vi "PID.vi"(6 "Reset I?":bool, 7 "permissable error range":dbl, 9 "Loop Period":dbl, 10 "Gains":cluster{"kP":dbl, "kI":dbl, "kD":dbl}, 11 "Error":dbl format="%#_13g") -> (1 "PID Variables":cluster{"P":dbl, "I":dbl, "D":dbl, "P+I+D":dbl}, 2 "Device has arrived":bool, 3 "Output":dbl)   [LabVIEW 2015]
uses:
  <vilib>/Analysis/3filter.llb/Filter Passband Type.ctl
  <vilib>/ptbypt/NI_PtbyPt.lvlib
  <vilib>/Analysis/NI_AALBase.lvlib
panel:
  in  "I_Cap":dbl=1.0
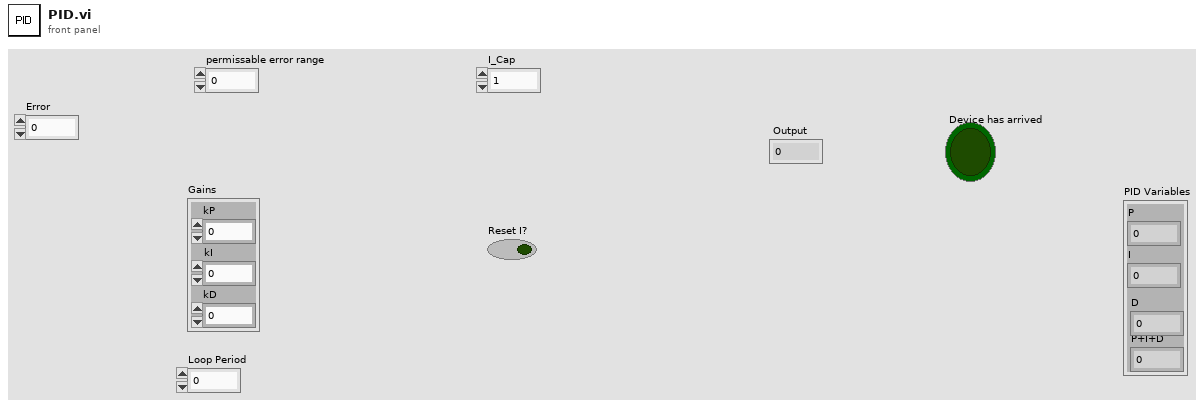
[diagram p1: front panel]
types:
  T1 = typedef "NI_AALBase.lvlib/Filter Passband Type.ctl" = enum32{"Lowpass", "Highpass", "Bandpass", "Bandstop"}
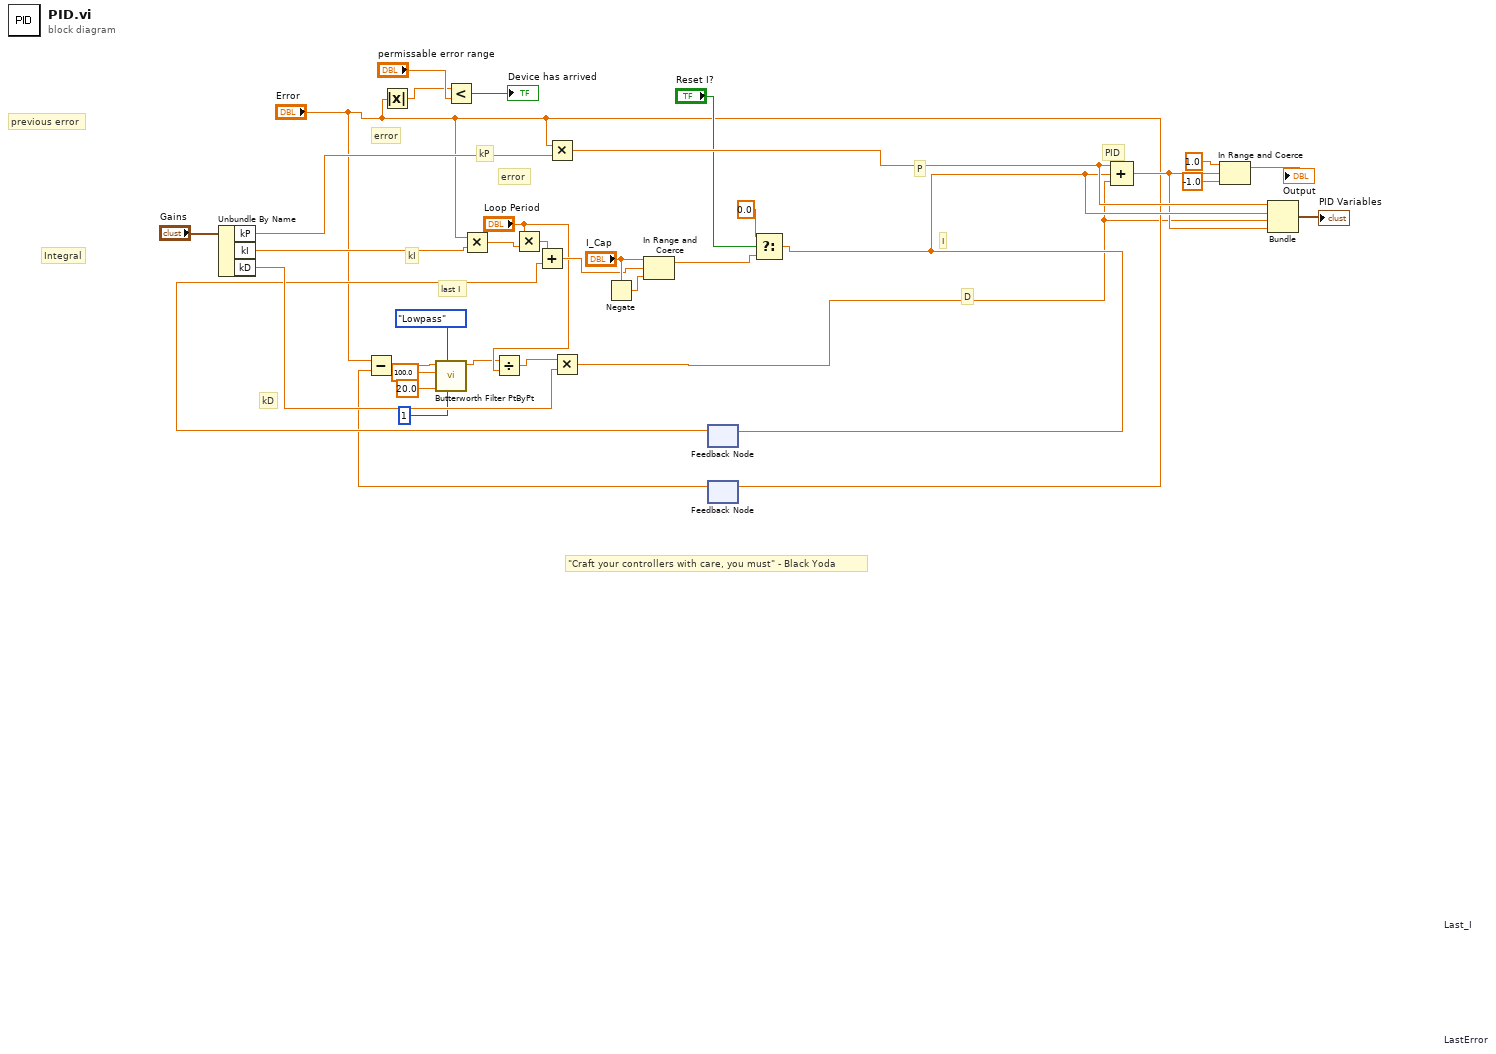
[diagram p0: block diagram]
diagram:
  # "last I"
  # "kI"
  # "error"
  # "kD"
  # "kP"
  # "error"
  # "PID"
  # "D"
  # "I"
  # "P"
  # "Integral"
  # "previous error"
  # "\"Craft your controllers with care, you must\" - Black Yoda"
  n1 = Unbundle By Name("Gains") -> ("kP"=w33:dbl, "kI"=w31:dbl, "kD"=w32:dbl)
  n2 = Absolute Value(x="Error") -> (abs(x)=w16:dbl)
  n3 = Less?(x=w16, y="permissable error range") -> (x < y?=→"Device has arrived":bool)
  n4 = Multiply(x="Error", y=w31) -> (x*y=w17:dbl)
  n5 = Multiply(x="Loop Period", y=w17) -> (x*y=w18:dbl)
  n6 = Multiply(x="Error", y=w33) -> (x*y=w13:dbl)
  n7 = Negate(x="I_Cap") -> (-x=w30:dbl)
  n8 = feedback #1 "Last_I"() -> (w23:dbl)  [unwired: 1 in]
  n9 = Add(x=w18, y=w23) -> (x+y=w26:dbl)
  n10 = In Range and Coerce(upper limit="I_Cap", x=w26, lower limit=w30) -> (coerced(x)=w28:dbl)  [unwired: 1 out]
  n11 = feedback #2 "LastError"() -> (w22:dbl)  [unwired: 1 in]
  n12 = Subtract(x="Error", y=w22) -> (x-y=w7:dbl)
  n13 = call <vilib>:"Butterworth Filter PtByPt.vi"("order"=1, "filter type"=Filter_Passband_Type."Lowpass", "low cutoff freq: fl"=20.0, "sampling freq: fs"=100.0, "x"=w7) -> ("Filtered x"=w8:dbl)  [unwired: 4 in, 1 out]
  n14 = Divide(x=w8, y="Loop Period") -> (x/y=w14:dbl)
  n15 = Multiply(x=w14, y=w32) -> (x*y=w1:dbl)
  n16 = feedback-in #2("Error") -> ()
  n17 = Select(t=0.0, s="Reset I?", f=w28) -> (s? t:f=w12:dbl)
  n18 = feedback-in #1(w12) -> ()
  n19 = Compound Arithmetic op=ADD(w13, w12, w1) -> (w11:dbl)
  n20 = In Range and Coerce(upper limit=1.0, x=w11, lower limit=-1.0) -> (coerced(x)=→"Output":dbl)  [unwired: 1 out]
  n21 = Bundle(w13, "I_Cap"=w12, w1, w11) -> (→"PID Variables":cluster{dbl, "I_Cap":dbl, dbl, dbl})  [unwired: 1 in]
